vi "Block Processing.vi"(4 "averaging parameters":T4={"averaging mode"=enum."No averaging", "weighting mode"=enum."Exponential", "number of averages"=10, "linear mode"=enum."One shot"}, 6 "window and overlap":cluster{"window":u32, "overlap":dbl}={"window"=1, "overlap"=32.0} {"window" items=["None "=0, "Hanning"=1, "Flat Top"=6, "7 Term B-Harris"=8]}, 7 "measure call context":refnum<class "Measure Call Context.lvclass">, 10 "DAQmx Configuration":T1 {"Run Mode" items=["Run Once", "Continuously"]; "Block Size" min=0; "Sample Rate (Hz)" min=0.0; "Trigger Type" items=["None", "Analog Reference"]; "Channel Table"."input terminal configuration" items=["default"=-1, "RSE"=10083, "NRSE"=10078, "Differential"=10106, "Pseudodifferential"=12529]; "Channel Table"."Channel Type" items=["Voltage (V)"=0, "Charge (C)"=9, "-"=99, "SPL (Pa)"=3, "Force (lbf)"=6, "Force (N)"=1, "Acceleration (g) - IEPE"=2, "Acceleration (g) - Charge"=12, "Acceleration (g) - 4 wire DC Voltage"=22, "Velocity (in/s)"=7, "Velocity (mm/s)"=8, "Prox Probe (mil)"=4, "Prox Probe (mm)"=5]}, 11 "data to process":T5) -> (0 "error out":errorcluster, 2 "last measurement results":T3)   [LabVIEW 2024, in "DSA_CFG_ACQ.lvlib"]
doc: "This VI reads and processes data from the Waveform Data Buffer, computes the averaged FFT, and pushes block results to the Global Data.Time Waveform Array and Global Data.Complex Spectra Array."
uses:
  DSA_CFG_ACQ.lvlib
  <extravilib>/ChannelInstances/Messenger-a[.](wfm(dbl))/))Channel.ctl
  <vilib>/Plug-In SDKs/Measurements/Measure Call Context/Measure Call Context.lvclass
  <vilib>/Addons/_XControls/Numeric with String Overlay/Numeric with String Overlay.xctl
  Dynamic Signal Acquisition (Interactive) UI/SFPConfiguration_1700.ctl
  <vilib>/addons/_NISVFA/_Shared subVIs/Controls/svc_Window.ctl
  Dynamic Signal Acquisition (Interactive) UI/SFPDAQ Configuration.ctl
  Dynamic Signal Acquisition (Interactive) UI/SFPDAQmx Channel Info.ctl
  subVIs/Message Queue/Message Cluster.ctl
  subVIs/SFPBlock Processing Loop State Manager.vi/8ab9d2bb-6bd8-408b-a319-3e4023a23bad.vi
  <extravilib>/ChannelInstances/Messenger-a[.](wfm(dbl))/Endpoint.vi
  <vilib>/addons/_NISVFA/_Baseband FFT/SVFA Power Spectrum (N Ch).vi
  subVIs/Message Queue/SFPMessage Queue.lvlib
  Dynamic Signal Acquisition (Interactive) UI/Dynamic Signal Acquisition (Interactive) UI.lvlib
  <extravilib>/ChannelInstances/Messenger-a[.](wfm(dbl)).lvlib
  <vilib>/addons/_NISVFA/_Shared subVIs/Data Objects/Waveforms (DBL)/Waveforms (N Ch).lvclass
  Measurement Results.ctl
  Dynamic Signal Acquisition (Interactive).lvlib
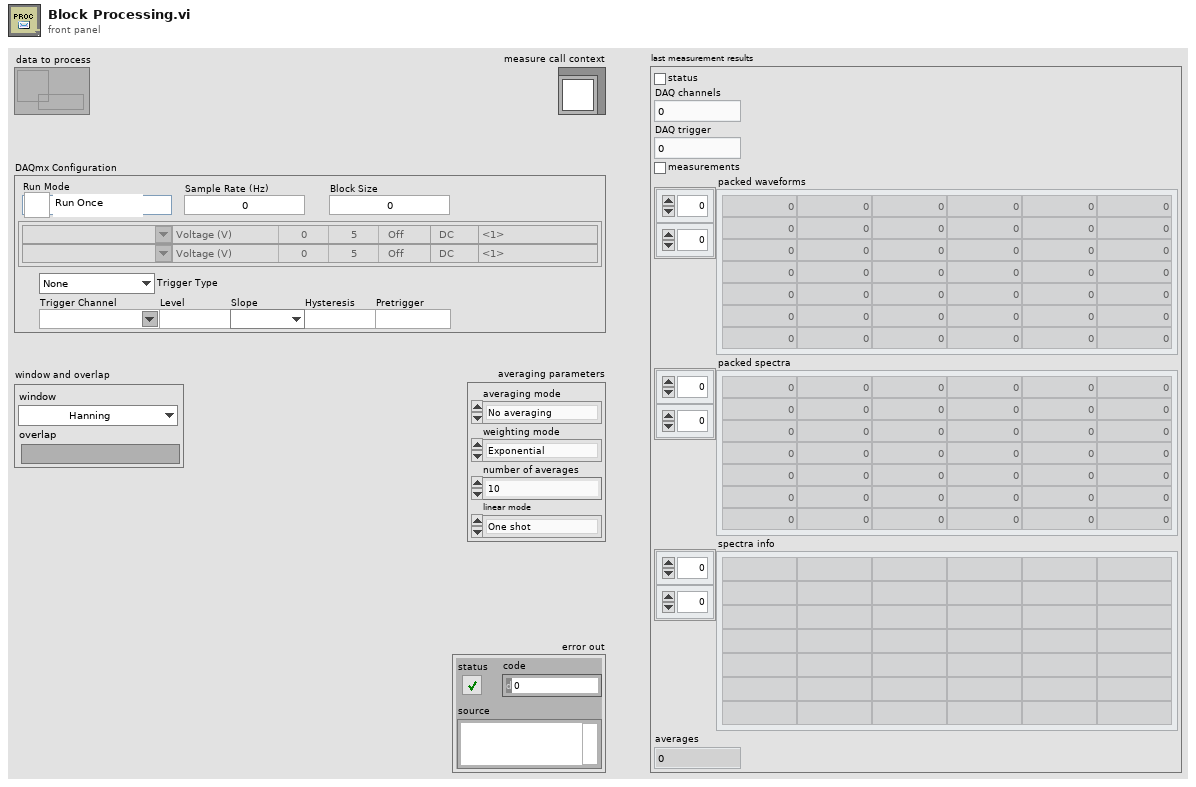
[diagram p1: front panel]
types:
  T1 = typedef "Dynamic Signal Acquisition (Interactive) UI.lvlib/SFPDAQ Configuration.ctl" = cluster{"Run Mode":u16, "Sample Rate (Hz)":dbl, "Block Size":i32, "Channel Table":T2[], "Trigger Type":u16, "Trigger Channel":string, "Level":dbl, "Pretrigger":i32, "Hysteresis":dbl, "Slope":enum16{"Falling", "Rising"}}
  T2 = typedef "Dynamic Signal Acquisition (Interactive) UI.lvlib/SFPDAQmx Channel Info.ctl" = cluster{"DAQmx Channel":tag, "Channel Type":u16, "Max":dbl, "Sensitivity":dbl, "Coupling":enum16{"AC", "DC"}, "input terminal configuration":i32, "excitation":enum16{"Off", "Min", "Max"}}
  T3 = typedef "Dynamic Signal Acquisition (Interactive).lvlib/Measurement Results.ctl" = cluster{"status":bool, "DAQ channels":u32, "DAQ trigger":u32, "measurements":bool, "packed waveforms":dbl[][], "packed spectra":dbl[][], "spectra info":string[][], "averages":dbl}
  T4 = cluster{"averaging mode":enum16{"No averaging", "Vector averaging", "RMS averaging", "Peak hold"}, "weighting mode":enum16{"Linear", "Exponential"}, "number of averages":u32, "linear mode":enum16{"One shot", "Auto restart"}}
  T5 = typedef "Messenger-a[.](wfm(dbl)).lvlib/))Channel.ctl" = refnum<queue>
  T6 = typedef "DSA_CFG_ACQ.lvlib/SFPMessage Queue.lvlib/Message Cluster.ctl" = cluster{"Message":string, "Message Data":variant}
  T7 = typedef "Dynamic Signal Acquisition (Interactive) UI.lvlib/SFPConfiguration_1700.ctl" = cluster{"version":string, "source":string, "Global Configuration":cluster{"directory":path, "operator":string, "comments":string, "Ref Ch":string}, "Wfm Subset":cluster{"Measure on waveform subset":bool, "waveform subset":cluster{"start index":i32, "length":i32}}, "FFT":cluster{"window":T8, "desired scaling":cluster{"linear or dB":enum16{"no change", "linear", "dB"}, "dB reference":dbl, "power or magnitude":enum16{"no change", "power", "magnitude"}, "view":enum16{"no change", "rms", "peak", "peak-peak"}}, "spectral density desired":enum16{"no change", "spectrum", "spectral density"}, "frequency range":cluster{"start":dbl, "stop":dbl}, "overlap":dbl, "averaging parameters":cluster{"averaging mode":enum16{"No averaging", "Vector averaging", "RMS averaging", "Peak hold"}, "weighting mode":enum16{"Linear", "Exponential"}, "number of averages":u32, "linear mode":enum16{"One shot", "Auto restart"}}}, "DAQ Config":T1, "logging duration":dbl, "Font Size":u16, "BG Color":u32}
  T8 = typedef "svc_Window.ctl" = u32
  T9 = cluster{"reset":bool, "read mode":enum16{"Last", "Continuous", "Overlapping"}, "read timeout":i32, "Measure delay":dbl, "time stamp":timestamp, "Configuration":T7}
  T10 = enum16{"No averaging", "Vector averaging", "RMS averaging", "Peak hold"}
  T11 = typedef "svc_Spectrum Info.ctl" = cluster{"channel name":string, "description":string, "x-axis units":T12, "spectral info":cluster{"spectrum type":T13, "linear/dB":enum16{"linear", "dB"}, "window":u16, "window size":i32, "FFT size":i32}, "engineering units":T14, "custom label":string, "dB reference [EU]":dbl, "peak units":enum16{"rms", "peak", "peak-peak"}, "weighting filter":T15, "spectral density?":bool, "unit label":string, "spectrum skewed?":bool, "complimentary spectrum units":T16}
  T12 = typedef "svc_X-Axis Units.ctl" = u16
  T13 = typedef "svc_Spectrum Type.ctl" = enum16{"FFT Spectrum [complex]", "Amplitude [Magnitude]", "Power [Magnitude^2]", "Cross Spectrum [complex]", "Frequency Response [Complex]"}
  T14 = typedef "svc_Engineering Units Text Ring.ctl" = u16
  T15 = typedef "svc_Weighting Filter Text Ring.ctl" = u16
  T16 = typedef "svc_Complimentary Spectrum Units.ctl" = enum16{"none", "radians", "degrees", "cycles", "imaginary"}
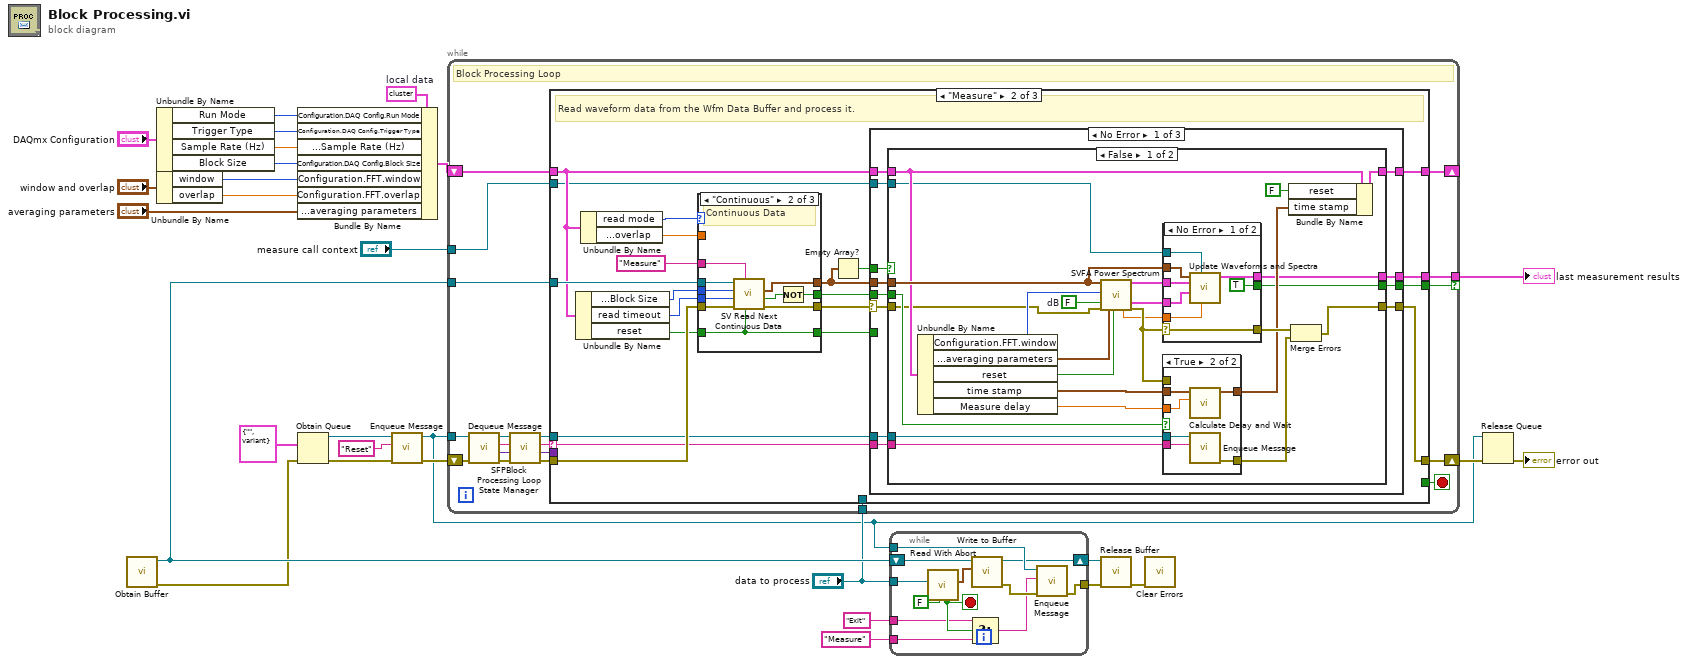
[diagram p0: block diagram]
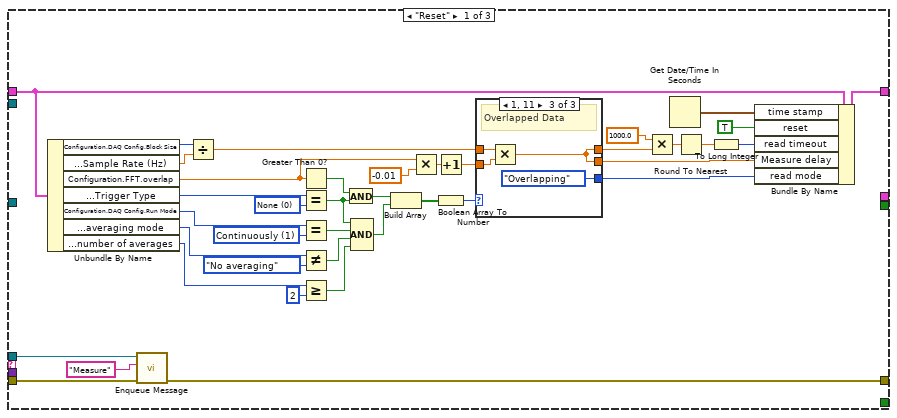
[diagram p2: hidden frame]
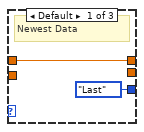
[diagram p3: hidden frame]
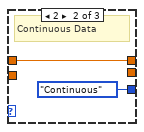
[diagram p4: hidden frame]
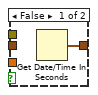
[diagram p6: hidden frame]
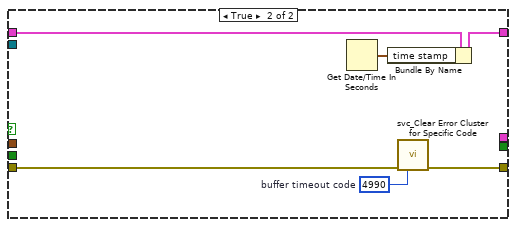
[diagram p7: hidden frame]
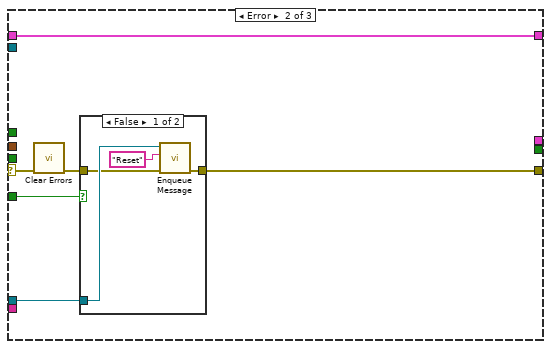
[diagram p8: hidden frame]
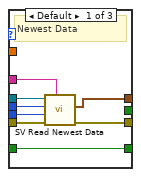
[diagram p11: hidden frame]
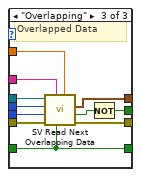
[diagram p12: hidden frame]
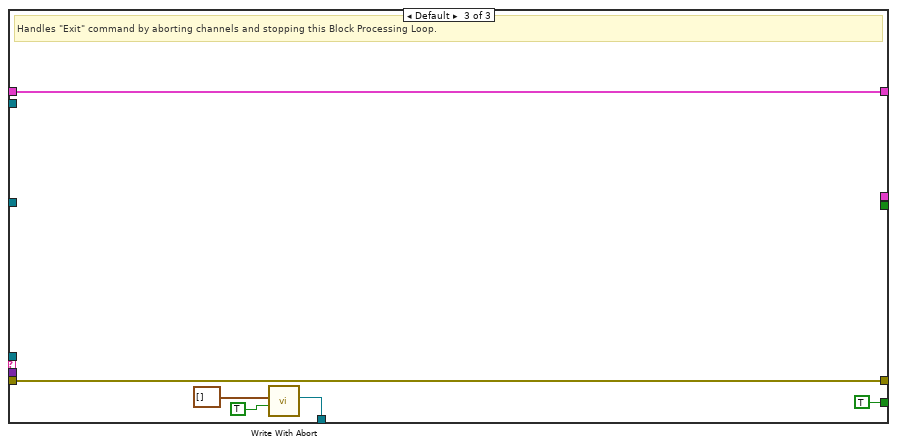
[diagram p13: hidden frame]
diagram:
  w29 = T9 {"reset"=TRUE, "read mode"=enum."Overlapping", "read timeout"=0, "Measure delay"=0.0, "time stamp"=timestamp(0 s since 1904-01-01), "Configuration"={"version"="", "source"="", "Global Configuration"={"directory"=path "", "operator"="", "comments"="", "Ref Ch"=""}, "Wfm Subset"={"Measure on waveform subset"=FALSE, "waveform subset"={"start index"=0, "length"=0}}, "FFT"={"window"=0, "desired scaling"={"linear or dB"=enum."no change", "dB reference"=0.0, "power or magnitude"=enum."no change", "view"=enum."no change"}, "spectral density desired"=enum."no change", "frequency range"={"start"=20.0, "stop"=20000.0}, "overlap"=50.0, "averaging parameters"={"averaging mode"=enum."No averaging", "weighting mode"=enum."Exponential", "number of averages"=10, "linear mode"=enum."One shot"}}, "DAQ Config"={"Run Mode"=0, "Sample Rate (Hz)"=51200.0, "Block Size"=5120, "Channel Table"=[{"DAQmx Channel"="", "Channel Type"=0, "Max"=0.0, "Sensitivity"=5.0, "Coupling"=enum."DC", "input terminal configuration"=1, "excitation"=enum."Off"}], "Trigger Type"=0, "Trigger Channel"="", "Level"=0.0, "Pretrigger"=20, "Hysteresis"=0.0, "Slope"=enum."Rising"}, "logging duration"=0.0, "Font Size"=15, "BG Color"=16728830}}  # local data
  n1 = call <vilib>:"Obtain Buffer.vi"() -> ("error out"=w21:errorcluster, "buffer out"=w23:refnum<data-value>)  [unwired: 10 in]
  n2 = Unbundle By Name("DAQmx Configuration") -> ("Run Mode"=w4:u16, "Trigger Type"=w3:u16, "Sample Rate (Hz)"=w2:dbl, "Block Size"=w1:i32)
  n3 = Unbundle By Name("window and overlap") -> ("window"=w12:u32, "overlap"=w11:dbl)
  n4 = Bundle By Name(cluster=w29, "Configuration.DAQ Config.Run Mode"=w4, "Configuration.DAQ Config.Trigger Type"=w3, "Configuration.DAQ Config.Sample Rate (Hz)"=w2, "Configuration.DAQ Config.Block Size"=w1, "Configuration.FFT.window"=w12, "Configuration.FFT.overlap"=w11, "Configuration.FFT.averaging parameters"="averaging parameters") -> (w28:T9)
  n5 = Obtain Queue(element data type=T6 {"Message"="", "Message Data"=variant} ("Message Cluster"), error in (no error)=w21) -> (queue out=w17:refnum<queue>, error out=w16:errorcluster)  [unwired: 3 in, 1 out]
  n6 = call "Enqueue Message.vi"("error in"=w16, "message"="Reset" ("Message"), "message queue"=w17) -> ("error out"=w15:errorcluster, "dup message queue"=w14:refnum<queue>)  [unwired: 7 in]
  n7 = while "BLOCK PROCESSING and DISPLAY UPDATES: Managed Action Engine that Consumes Block Data and Performs Actions such as Measure, Save, Load, and Update Graph" {
    tunnel: w14 -> [w36]
    shift-right: [w47] -> w26
    shift-left: w15 -> [w46]
    shift-right: [w37] -> _
    shift-left: w28 -> [w38]
    tunnel: w23 -> [w35]
    tunnel: "data to process" -> [w34]
    tunnel: "measure call context" -> [w33]
    tunnel: [w31] -> w7 if=w30
    stop <- w48 stop-if-true
    # "Block Processing Loop"
    n8 = call "Dequeue Message.vi"("error in"=w46, "message queue"=w36) -> ("error out"=w41:errorcluster, "Message Data"=w42:variant, "Message"=w43:string, "dup message queue"=w45:refnum<queue>)  [unwired: 6 in]
    n9 = call "SFPBlock Processing Loop State Manager.vi"("error in"=w41, "variant"=w42, "message in"=w43, "Message Queue"=w45) -> ("error out"=w40:errorcluster, "duplicate variant"=w39:variant, "message out"=w32:string, "duplicate Message Queue"=w44:refnum<queue>)  [unwired: 4 in]
    n10 = case shown="\"Measure\"" w32 {
      selector: w32 -> [_ w111 _]
      tunnel: [_ _ TRUE] -> w48
      tunnel: w40 -> [w62 w115 w219]
      tunnel: [w61 w116 w219] -> w47
      tunnel: w44 -> [w63 w112 _]
      tunnel: w39 -> [_ _ _]
      tunnel: w38 -> [w50 w102 w223]
      tunnel: [w49 w103 w223] -> w37
      tunnel: w35 -> [_ w106 _]
      tunnel: [_ _ w221] -> w34
      tunnel: w33 -> [_ w98 _]
      tunnel: [_ w97 _] -> w31
      tunnel: [_ w96 _] -> w30
      frame "Reset" {
        w85 = u16 1 items=["Run Once", "Continuously"] ("Run Mode")
        w87 = u16 0 items=["None", "Analog Reference"] ("Trigger Type")
        n11 = Unbundle By Name(w50) -> ("Configuration.DAQ Config.Block Size"=w67:i32, "Configuration.DAQ Config.Sample Rate (Hz)"=w72:dbl, "Configuration.FFT.overlap"=w56:dbl, "Configuration.DAQ Config.Trigger Type"=w77:u16, "Configuration.DAQ Config.Run Mode"=w86:u16, "Configuration.FFT.averaging parameters.averaging mode"=w83:T10, "Configuration.FFT.averaging parameters.number of averages"=w66:u32)
        n12 = call "Enqueue Message.vi"("error in"=w62, "message"="Measure" ("Message"), "message queue"=w63) -> ("error out"=w61:errorcluster)  [unwired: 7 in, 1 out]
        n13 = Divide(x=w67, y=w72) -> (x/y=w73:dbl)
        n14 = Greater Than 0?(x=w56) -> (x > 0?=w75:bool)
        n15 = Equal?(x=w77, y=w87) -> (x = y?=w68:bool)
        n16 = Equal?(x=w86, y=w85) -> (x = y?=w82:bool)
        n17 = Not Equal?(x=w83, y=T10."No averaging" ("averaging mode")) -> (x != y?=w81:bool)
        n18 = Greater Or Equal?(x=w66, y=u32 2) -> (x >= y?=w80:bool)
        n19 = And(x=w75, y=w68) -> (x .and. y?=w76:bool)
        n20 = Compound Arithmetic op=AND(w68, w82, w81, w80) -> (w79:bool)
        n21 = Build Array(w76, w79) -> (w78:bool[])
        n22 = Multiply(x=w56, y=-0.01) -> (x*y=w59:dbl)
        n23 = Increment(x=w59) -> (x+1=w57:dbl)
        n24 = Boolean Array To Number(Boolean array=w78) -> (number=w74:u32)
        n25 = case shown="1, 11" w74 {
          tunnel: w73 -> [w88 w90 w95]
          tunnel: [enum16{"Last", "Continuous", "Overlapping"}."Last" ("read mode") enum16{"Last", "Continuous", "Overlapping"}."Continuous" ("read mode") enum16{"Last", "Continuous", "Overlapping"}."Overlapping" ("read mode")] -> w70
          tunnel: [_ _ w92] -> w54
          tunnel: w57 -> [_ _ w93]
          tunnel: [w88 w90 w92] -> w53
          frame Default {
            # "Newest Data"
          }
          frame 2 {
            # "Continuous Data"
          }
          frame 1, 3 {
            # "Overlapped Data"
            n26 = Multiply(x=w95, y=w93) -> (x*y=w92:dbl)
          }
        }
        n27 = Multiply(x=1000.0, y=w53) -> (x*y=w55:dbl)
        n28 = Get Date/Time In Seconds() -> (seconds since 1Jan1904=w60:timestamp)
        n29 = Round To Nearest(number=w55) -> (nearest integer value=w51:dbl)
        n30 = To Long Integer(number=w51) -> (32bit integer=w69:i32)
        n31 = Bundle By Name(cluster=w50, "time stamp"=w60, "reset"=TRUE, "read timeout"=w69, "Measure delay"=w54, "read mode"=w70) -> (w49:T9)
      }
      frame "Measure" {
        # "Read waveform data from the Wfm Data Buffer and process it."
        n32 = Unbundle By Name(w102) -> ("Configuration.DAQ Config.Block Size"=w107:i32, "read timeout"=w104:i32, "reset"=w105:bool)
        n33 = Unbundle By Name(w102) -> ("read mode"=w101:enum16{"Last", "Continuous", "Overlapping"}, "Configuration.FFT.overlap"=w100:dbl)
        n34 = case shown="\"Continuous\"" w101 {
          tunnel: w106 -> [w196 w206 w217]
          tunnel: [w195 w205 w216] -> w113
          tunnel: [w194 w204 w215] -> w109
          tunnel: w115 -> [w193 w203 w214]
          tunnel: w107 -> [w192 w202 w213]
          tunnel: w100 -> [_ _ w208]
          tunnel: "Measure" ("reader ID") -> [w191 w201 w212]
          tunnel: w105 -> [w189 w197 w207]
          tunnel: [_ w198 w210] -> w110
          tunnel: w104 -> [w190 w200 w209]
          tunnel: [w189 w197 w207] -> w99
          frame Default {
            # "Newest Data"
            n35 = call <vilib>:"SV Read Newest Data.vi"("reader ID"=w191, "error in (no error)"=w193, "timeout (0 ms)"=w190, "block length (-1 = all)"=w192, "buffer"=w196) -> ("error out"=w195:errorcluster, "waveforms subset"=w194:waveform(dbl)[])  [unwired: 3 in, 2 out]
          }
          frame "Continuous" {
            # "Continuous Data"
            n36 = call <vilib>:"SV Read Next Continuous Data.vi"("reset start (F)"=w197, "reader ID"=w201, "error in (no error)"=w203, "timeout (0 ms)"=w200, "block length (-1 = all)"=w202, "buffer"=w206) -> ("error out"=w205:errorcluster, "end of buffer"=w199:bool, "waveforms subset"=w204:waveform(dbl)[])  [unwired: 2 in, 1 out]
            n37 = Not(x=w199) -> (.not. x?=w198:bool)
          }
          frame "Overlapping" {
            # "Overlapped Data"
            n38 = call <vilib>:"SV Read Next Overlapping Data.vi"("overlap (50 %)"=w208, "reset start (F)"=w207, "reader ID"=w212, "error in (no error)"=w214, "timeout (0 ms)"=w209, "block length (4096 samples)"=w213, "buffer"=w217) -> ("error out"=w216:errorcluster, "end of buffer"=w211:bool, "waveforms subset"=w215:waveform(dbl)[])  [unwired: 1 in, 1 out]
            n39 = Not(x=w211) -> (.not. x?=w210:bool)
          }
        }
        n40 = Empty Array?(array=w109) -> (empty?=w108:bool)
        n41 = case shown="No Error" w113 {
          selector: w113 -> [w127 w180 w188]
          tunnel: w109 -> [w122 _ _]
          tunnel: [w128 w177 w188] -> w116
          tunnel: w112 -> [w126 w181 _]
          tunnel: w111 -> [w125 _ _]
          tunnel: w110 -> [w124 _ _]
          tunnel: w108 -> [w123 _ _]
          tunnel: w102 -> [w121 w179 w187]
          tunnel: [w120 w179 w187] -> w103
          tunnel: w99 -> [_ w176 _]
          tunnel: w98 -> [w119 _ _]
          tunnel: [w118 _ _] -> w97
          tunnel: [w117 _ _] -> w96
          frame No Error {
            n42 = case shown="False" w123 {
              tunnel: [w153 w173] -> w128
              tunnel: w127 -> [w131 w174]
              tunnel: w122 -> [w152 _]
              tunnel: w126 -> [w151 _]
              tunnel: w125 -> [w150 _]
              tunnel: w124 -> [w144 _]
              tunnel: w121 -> [w134 w171]
              tunnel: [w143 w170] -> w120
              tunnel: w119 -> [w132 _]
              tunnel: [w130 _] -> w118
              tunnel: [w129 _] -> w117
              frame False {
                w147 = FALSE  # dB
                n43 = Unbundle By Name(w134) -> ("Configuration.FFT.window"=w135:T8, "Configuration.FFT.averaging parameters"=w136:T4, "reset"=w137:bool, "time stamp"=w139:timestamp, "Measure delay"=w138:dbl)
                n44 = call-poly <vilib>:"SVFA Power Spectrum.vi"("scaled signals [EU]"=w152, "window"=w135, "dB On (T)"=w147, "error in (no error)"=w131, "averaging parameters"=w136, "restart averaging (F)"=w137) -> ("averages completed"=w133:dbl, "power spectra [dB EU]"=w148:cluster{"f0":dbl, "df":dbl, "magnitude":dbl[]}[], "spectrum info"=w140:T11[], "error out"=w146:errorcluster)  [unwired: 8 in, 2 out]
                n45 = case shown="No Error" w146 {
                  selector: w146 -> [w161 w162]
                  tunnel: w152 -> [w160 _]
                  tunnel: w148 -> [w159 _]
                  tunnel: w140 -> [w158 _]
                  tunnel: [w161 w162] -> w145
                  tunnel: w133 -> [w157 _]
                  tunnel: w132 -> [w156 _]
                  tunnel: [w155 _] -> w130
                  tunnel: [TRUE _] -> w129
                  frame No Error {
                    n46 = call "Update Waveforms and Spectra.vi"("averages completed"=w157, "measure call context in"=w156, "spectrum info"=w158, "power spectra [dB EU]"=w159, "waveforms subset"=w160) -> ("last measurement results"=w155:T3)  [unwired: 6 in]
                  }
                  frame Error {
                  }
                }
                n47 = case shown="True" w144 {
                  tunnel: w151 -> [_ w169]
                  tunnel: w150 -> [_ w166]
                  tunnel: [_ w168] -> w149
                  tunnel: w146 -> [_ _]
                  tunnel: w138 -> [_ w164]
                  tunnel: w139 -> [_ w165]
                  tunnel: [w163 w167] -> w142
                  frame False {
                    n48 = Get Date/Time In Seconds() -> (seconds since 1Jan1904=w163:timestamp)
                  }
                  frame True {
                    n49 = call "Calculate Delay and Wait.vi"("expected interval (s)"=w164, "previous time stamp"=w165) -> ("new time stamp"=w167:timestamp)  [unwired: 7 in]
                    n50 = call "Enqueue Message.vi"("message"=w166, "message queue"=w169) -> ("error out"=w168:errorcluster)  [unwired: 8 in, 1 out]
                  }
                }
                n51 = Bundle By Name(cluster=w134, "reset"=FALSE, "time stamp"=w142) -> (w143:T9)
                n52 = Merge Errors(w145, w149) -> (w153:errorcluster)
              }
              frame True {
                w175 = 4990  # buffer timeout code
                n53 = Get Date/Time In Seconds() -> (seconds since 1Jan1904=w172:timestamp)
                n54 = Bundle By Name(cluster=w171, "time stamp"=w172) -> (w170:T9)
                n55 = call <vilib>:"svc_Clear Error Cluster for Specific Code.vi"("error in (no error)"=w174, "code"=w175) -> ("error out"=w173:errorcluster)  [unwired: 12 in, 1 out]
              }
            }
          }
          frame Error {
            n56 = call <vilib>:"Clear Errors.vi"("error in (no error)"=w180) -> ("error out"=w178:errorcluster)  [unwired: 5 in, 1 out]
            n57 = case shown="False" w176 {
              tunnel: w181 -> [w185 _]
              tunnel: w178 -> [w184 w186]
              tunnel: [w182 w186] -> w177
              frame False {
                n58 = call "Enqueue Message.vi"("error in"=w184, "message"="Reset" ("Message"), "message queue"=w185) -> ("error out"=w182:errorcluster)  [unwired: 7 in, 1 out]
              }
              frame True {
              }
            }
          }
          frame Default {
          }
        }
      }
      frame Default {
        # "Handles \"Exit\" command by aborting channels and stopping this Block Processing Loop."
        n59 = call <extravilib>:"Write With Abort.vi"("abort (F)"=TRUE, "element"=waveform(dbl)[] []) -> ("channel"=w221:T5)  [unwired: 6 in, 3 out]
      }
    }
  }
  "last measurement results" <- w7
  n60 = while {
    tunnel: w14 -> [w232]
    tunnel: "data to process" -> [w235]
    shift-right: [w230] -> w24
    shift-left: w23 -> [w231]
    tunnel: [w228] -> w20
    tunnel: "Exit" ("Message") -> [w226]
    tunnel: "Measure" ("Message") -> [w225]
    stop <- w227 stop-if-true
    n61 = call <extravilib>:"Read With Abort.vi"("abort (F)"=FALSE, "channel"=w235) -> ("element"=w234:waveform(dbl)[], "aborted?"=w227:bool)  [unwired: 6 in, 2 out]
    n62 = Select(t=w226, s=w227, f=w225) -> (s? t:f=w224:string)
    n63 = call <vilib>:"Write to Buffer.vi"("waveforms"=w234, "buffer"=w231) -> ("error out"=w229:errorcluster, "buffer out"=w230:refnum<data-value>)  [unwired: 7 in, 1 out]
    n64 = call "Enqueue Message.vi"("error in"=w229, "message"=w224, "message queue"=w232) -> ("error out"=w228:errorcluster)  [unwired: 7 in, 1 out]
  }
  n65 = call <vilib>:"Release Buffer.vi"("error in (no error)"=w20, "buffer"=w24) -> ("error out"=w19:errorcluster)  [unwired: 9 in]
  n66 = call <vilib>:"Clear Errors.vi"("error in (no error)"=w19) -> ()  [unwired: 5 in, 2 out]
  n67 = Release Queue(queue=w14, error in (no error)=w26) -> (error out=→"error out":errorcluster)  [unwired: 1 in, 2 out]
